vi "Create Dynamical Model (Acceleration Controlled).vi"() -> ()   [LabVIEW 2020]
uses:
  Infrastructure/Dynamical System Model Definition.ctl
  Infrastructure/Model Types.ctl
panel:
  out "Holonomic Robot Dynamical System Model":T1
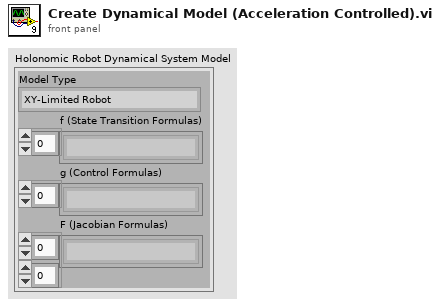
[diagram p1: front panel]
types:
  T1 = typedef "Dynamical System Model Definition.ctl" = cluster{"Model Type":T2, "f (State Transition Formulas)":string[], "g (Control Formulas)":string[], "F (Jacobian Formulas)":string[][]}
  T2 = typedef "Model Types.ctl" = enum16{"XY-Limited Robot", "Holonomic Robot (Acceleration Controlled)"}
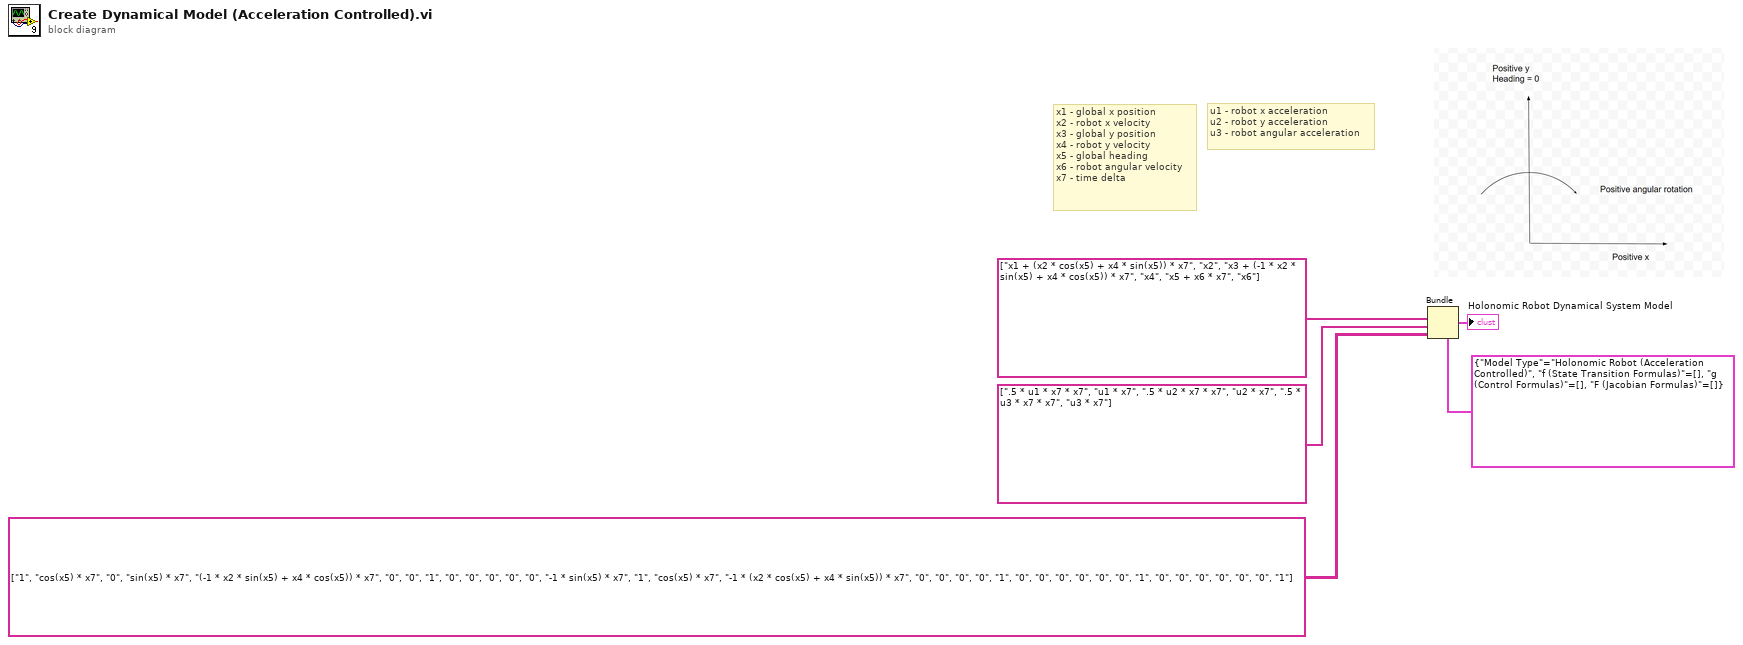
[diagram p0: block diagram]
diagram:
  # "u1 - robot x acceleration\nu2 - robot y acceleration\nu3 - robot angular acceleration"
  # "x1 - global x position\nx2 - robot x velocity\nx3 - global y position\nx4 - robot y velocity\nx5 - global heading\nx6 - robot angular velocity\nx7 - time delta"
  n1 = Bundle(cluster=T1 {"Model Type"=enum."Holonomic Robot (Acceleration Controlled)", "f (State Transition Formulas)"=[], "g (Control Formulas)"=[], "F (Jacobian Formulas)"=[]} ("Dynamical System Model Definition"), "f (State Transition Formulas)"=string[] ["x1 + (x2 * cos(x5) + x4 * sin(x5)) * x7", "x2", "x3 + (-1 * x2 * sin(x5) + x4 * cos(x5)) * x7", "x4", "x5 + x6 * x7", "x6"], "g (Control Formulas)"=string[] [".5 * u1 * x7 * x7", "u1 * x7", ".5 * u2 * x7 * x7", "u2 * x7", ".5 * u3 * x7 * x7", "u3 * x7"] ("f (State Transition Formulas)"), "F (Jacobian Formulas)"=string[][] [["1", "cos(x5) * x7", "0", "sin(x5) * x7", "(-1 * x2 * sin(x5) + x4 * cos(x5)) * x7", "0"], ["0", "1", "0", "0", "0", "0"], ["0", "-1 * sin(x5) * x7", "1", "cos(x5) * x7", "-1 * (x2 * cos(x5) + x4 * sin(x5)) * x7", "0"], ["0", "0", "0", "1", "0", "0"], ["0", "0", "0", "0", "1", "0"], ["0", "0", "0", "0", "0", "1"]]) -> (→"Holonomic Robot Dynamical System Model":T1)  [unwired: 1 in]
